vi "Loop Till Force Sensed Two Sensors.vi"(9 "Analog Input Pin 2":u8, 10 "Analog Input Pin":u8) -> (2 "Force Threshhold Reached":bool)   [LabVIEW 2013]
uses:
  <vilib>/Analysis/baseanly.llb/Mean (DBL).vi
  <vilib>/LabVIEW Interface for Arduino/LabVIEW Interface for Arduino.lvlib
  <vilib>/Analysis/NI_AALBase.lvlib
panel:
  out "Average Force":dbl(graph)
  out "Average Force":dbl
  out "Force2 Average":dbl format="%0.2f"
  out "Force vs Time 2":dbl(graph)
  out "Volatege vs Time 2":dbl(graph)
  out "Force1 Average":dbl format="%0.2f"
  out "Force vs Time":dbl(graph)
  out "Voltage Average":dbl format="%0.2f"
  in  "Array":dbl[](array[numeric])
  in  "Stop":bool
  out "Volatege vs Time":dbl(graph)
  out "output array":dbl[](array[numeric])
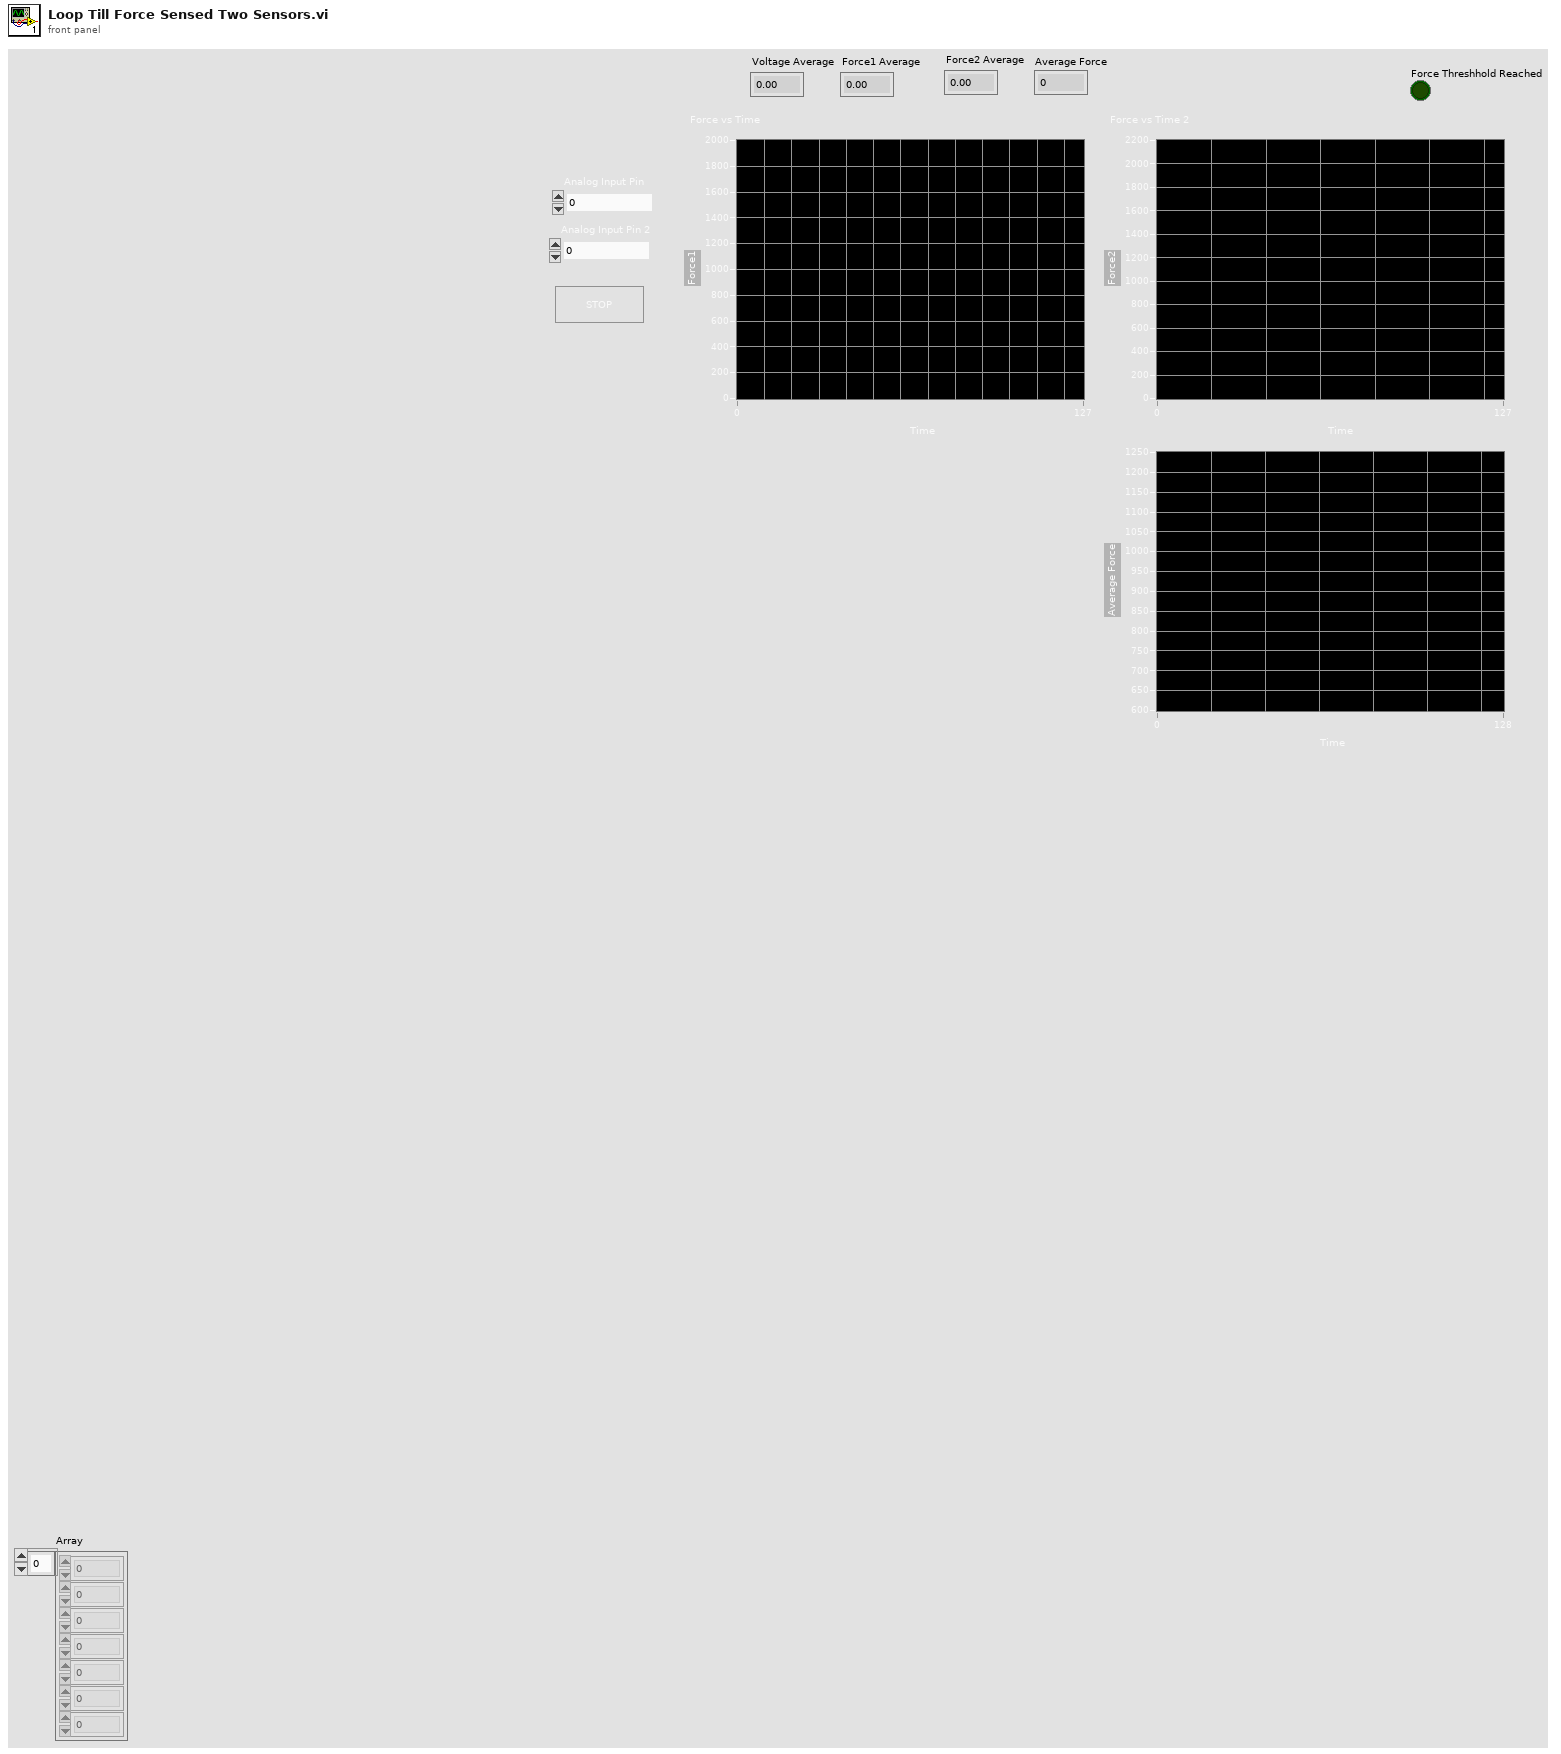
[diagram p1: front panel]
types:
  T1 = typedef "LabVIEW Interface for Arduino.lvlib/Arduino Resource.ctl" = cluster{"VISA resource":refnum<visa-resource-name>, "Board Type":T2, "Connection Type":enum8{"USB / Serial"}, "Bytes Per Packet (15)":u8}
  T2 = typedef "LabVIEW Interface for Arduino.lvlib/Board Type.ctl" = enum16{"Uno", "Dimuelanove w/Atmega 328", "Mega 2560"}
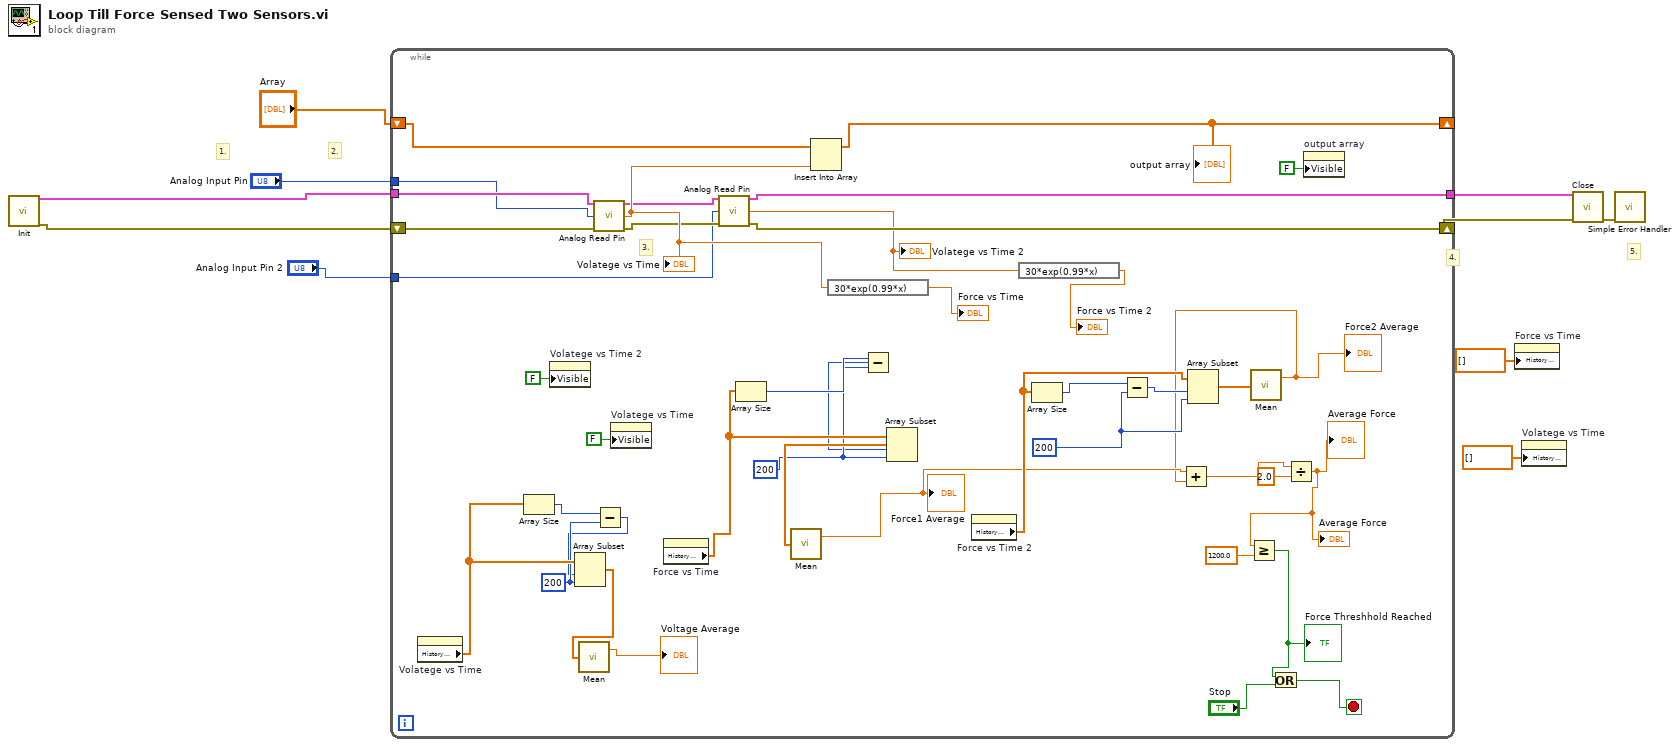
[diagram p0: block diagram]
diagram:
  # "5."
  # "4."
  # "2."
  # "1."
  n1 = call <vilib>:"Init.vi"() -> ("Arduino Resource"=w5:T1, "error out"=w3:errorcluster)  [unwired: 18 in]
  n2 = while {
    shift-right: [w24] -> w9
    shift-left: w3 -> [w29]
    shift-right: [w51] -> _
    shift-left: "Array" -> [w52]
    tunnel: w5 -> [w31]
    tunnel: "Analog Input Pin" -> [w30]
    tunnel: [w25] -> w2
    tunnel: "Analog Input Pin 2" -> [w26]
    stop <- w35 stop-if-true
    w17 = 200 ("length")
    w43 = 200 ("length")
    w40 = 200 ("length")
    # "3."
    n3 = property on="Volatege vs Time" class="WFChart (strict)"() -> ("History Data"=w47:dbl[])  [unwired: 2 in, 2 out]
    n4 = Array Size(array=w47) -> (size(s)=w44:i32)
    n5 = property on="Volatege vs Time 2" class="WFChart (strict)"("Visible"=FALSE) -> ()  [unwired: 2 in, 2 out]
    n6 = call <vilib>:"Analog Read Pin.vi"("Arduino Resource"=w31, "Analog Input Pin (0)"=w30, "error in"=w29) -> ("Arduino Resource"=w28:T1, "Voltage"=w32:dbl, "error out"=w27:errorcluster)  [unwired: 10 in]
    "Volatege vs Time" <- w32
    n7 = Subtract(x=w44, y=w43) -> (x-y=w42:i32)
    n8 = Array Subset(array=w47, index=w42, length=w43) -> (w45:dbl[])
    n9 = call-poly <vilib>:"Mean.vi"("X"=w45) -> ("mean"=→"Voltage Average":dbl)  [unwired: 1 out]
    n10 = property on="Volatege vs Time" class="WFChart (strict)"("Visible"=FALSE) -> ()  [unwired: 2 in, 2 out]
    n11 = property on="Force vs Time" class="WFChart (strict)"() -> ("History Data"=w49:dbl[])  [unwired: 2 in, 2 out]
    n12 = call <vilib>:"Analog Read Pin.vi"("Arduino Resource"=w28, "Analog Input Pin (0)"=w26, "error in"=w27) -> ("Arduino Resource"=w25:T1, "Voltage"=w23:dbl, "error out"=w24:errorcluster)  [unwired: 10 in]
    "Volatege vs Time 2" <- w23
    n13 = Array Size(array=w49) -> (size(s)=w41:i32)
    n14 = Insert Into Array(array=w52, new element=w32) -> (w51:dbl[])  [unwired: 1 in]
    "output array" <- w51
    n15 = expression code="30*exp(0.99*x)"(w32) -> (→"Force vs Time":dbl)
    n16 = Subtract(x=w41, y=w40) -> (x-y=w39:i32)
    n17 = Array Subset(array=w49, index=w39, length=w40) -> (w48:dbl[])
    n18 = call-poly <vilib>:"Mean.vi"("X"=w48) -> ("mean"=w13:dbl)  [unwired: 1 out]
    "Force1 Average" <- w13
    n19 = property on="Force vs Time 2" class="WFChart (strict)"() -> ("History Data"=w20:dbl[])  [unwired: 2 in, 2 out]
    n20 = expression code="30*exp(0.99*x)"(w23) -> (→"Force vs Time 2":dbl)
    n21 = Array Size(array=w20) -> (size(s)=w19:i32)
    n22 = Subtract(x=w19, y=w17) -> (x-y=w18:i32)
    n23 = Array Subset(array=w20, index=w18, length=w17) -> (w16:dbl[])
    n24 = call-poly <vilib>:"Mean.vi"("X"=w16) -> ("mean"=w12:dbl)  [unwired: 1 out]
    "Force2 Average" <- w12
    n25 = Add(x=w13, y=w12) -> (x+y=w14:dbl)
    n26 = Divide(x=w14, y=2.0) -> (x/y=w11:dbl)
    "Average Force" <- w11
    "Average Force" <- w11
    n27 = Greater Or Equal?(x=w11, y=1200.0) -> (x >= y?=w37:bool)
    "Force Threshhold Reached" <- w37
    n28 = Or(x=w37, y="Stop") -> (x .or. y?=w35:bool)
    n29 = property on="output array" class="Arr (strict)"("Visible"=FALSE) -> ()  [unwired: 2 in, 2 out]
  }
  n30 = property on="Force vs Time" class="WFChart (strict)"("History Data"=dbl[] []) -> ()  [unwired: 2 in, 2 out]
  n31 = property on="Volatege vs Time" class="WFChart (strict)"("History Data"=dbl[] []) -> ()  [unwired: 2 in, 2 out]
  n32 = call <vilib>:"Close.vi"("Arduino Resource"=w2, "error in"=w9) -> ("error out"=w10:errorcluster)  [unwired: 13 in]
  n33 = call <vilib>:"Simple Error Handler.vi"("error in (no error)"=w10) -> ()  [unwired: 4 in, 5 out]
